vi "Send Define Panel Actors to Display.vi"(7 "Message Priority (Normal)":T1=enum."Normal", 8 "error in (no error)":errorcluster, 10 "panelsEnQrs":refnum<class "Message Enqueuer.lvclass">[](array[class]), 11 "Message Enqueuer":refnum<class "Message Enqueuer.lvclass">) -> (0 "error out":errorcluster, 3 "Message Enqueuer out":refnum<class "Message Enqueuer.lvclass">)   [LabVIEW 2020, in "HSplitted.lvlib" / "Define Panel Actors to Display Msg 2.lvclass"]
doc: "This VI sends the message to an actor."
uses:
  Define Panel Actors to Display Msg 2.lvclass
  <vilib>/ActorFramework/Message Enqueuer/Message Enqueuer.lvclass
  <vilib>/ActorFramework/Message Enqueuer/Message Priority.ctl
  C:/Program Files (x86)/National Instruments/LabVIEW 2020/vi.lib/ActorFramework/Message/Message.lvclass
  Define Panel Actors to Display Msg 2.lvclass/Define Panel Actors to Display Msg 2.ctl
  <vilib>/ActorFramework/Message Enqueuer/Message Enqueuer.lvclass/Message Enqueuer.ctl
  <vilib>/ActorFramework/Message Priority Queue/Priority Enqueue.vi
  C:/Users/Test/Git/MGIPanelActors-Exploration/src/HSplitted/HSplitted Messages/Define Panel Actors to Display Msg/Define Panel Actors to Display Msg 2.lvclass
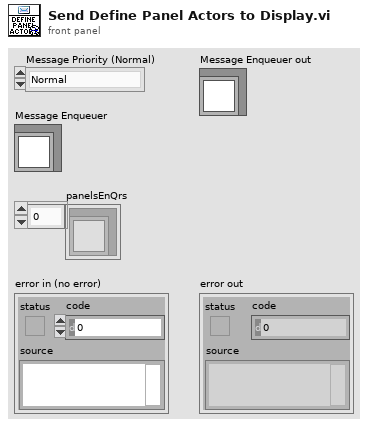
[diagram p1: front panel]
types:
  T1 = typedef "Actor Framework.lvlib/Message Enqueuer.lvclass/Message Priority.ctl" = enum16{"Low", "Normal", "High"}
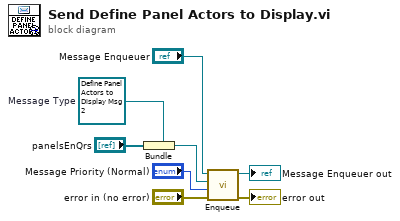
[diagram p0: block diagram]
diagram:
  w5 = refnum<class "Define Panel Actors to Display Msg 2.lvclass"> refnum  # Message Type
  n1 = Bundle(cluster=w5, "panelsEnQrs") -> (w4:refnum<class "Define Panel Actors to Display Msg 2.lvclass">)
  n2 = call <vilib>:"Enqueue.vi"("error in (no error)"="error in (no error)", "Message Priority (Normal)"="Message Priority (Normal)", "Message"=w4, "Message Enqueuer in"="Message Enqueuer") -> ("error out"=→"error out":errorcluster, "Message Enqueuer in"=→"Message Enqueuer out":refnum<class "Message Enqueuer.lvclass">)  [unwired: 6 in]
